vi "Index General Process Info.vi"(11 "process information":dbl[](array[numeric])) -> (1 "Process Memory Used (MB)":dbl, 2 "Process HandleCount":dbl, 3 "Process Thread Count":dbl)   [LabVIEW 2016]
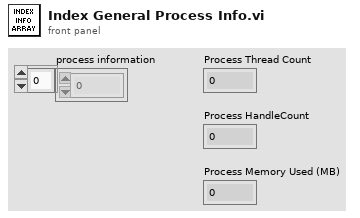
[diagram p1: front panel]
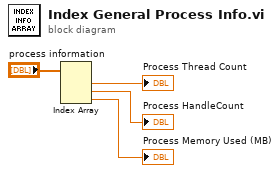
[diagram p0: block diagram]
diagram:
  n1 = Index Array(array="process information") -> (element #1=→"Process Thread Count":dbl, element #2=→"Process HandleCount":dbl, element #3=→"Process Memory Used (MB)":dbl)  [unwired: 3 in]
